vi "tcp_echo_client.vi"() -> ()   [LabVIEW 2015]
panel:
  out "good echo":bool
  out "message received":string
  in  "message to send":string="hello there.\r\n"
  out "available IP addresses":string[](array[string])
  in  "remote port or service name":u16=7
  in  "address":string
  # "try tcp ping"
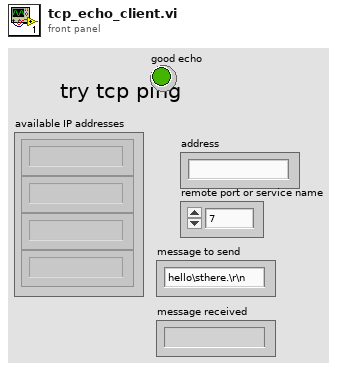
[diagram p1: front panel]
types:
  T1 = enum16{"Standard", "Buffered", "CRLF", "Immediate"}
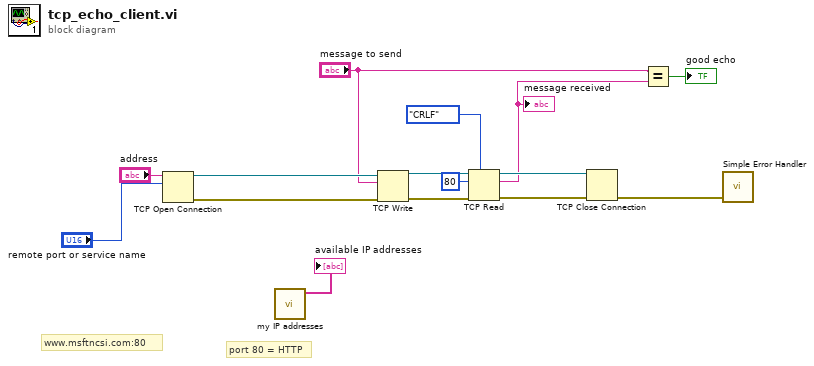
[diagram p0: block diagram]
diagram:
  # "port 80 = HTTP"
  # "www.msftncsi.com:80"
  n1 = TCP Open Connection(address="address", remote port or service name="remote port or service name") -> (connection ID=w4:refnum<k5>, error out=w5:errorcluster)  [unwired: 3 in]
  n2 = call "my IP addresses.vi"() -> ("available IP addresses"=→"available IP addresses":string[])  [unwired: 10 in, 1 out]
  n3 = TCP Write(connection ID=w4, data in="message to send", error in (no error)=w5) -> (connection ID out=w11:refnum<k5>, error out=w12:errorcluster)  [unwired: 1 in, 1 out]
  n4 = TCP Read(connection ID=w11, bytes to read=80, error in (no error)=w12, 7:T1."CRLF" ("mode (standard)")) -> (connection ID out=w8:refnum<k5>, data out=w3:string, error out=w9:errorcluster)  [unwired: 1 in]
  "message received" <- w3
  n5 = TCP Close Connection(connection ID=w8, error in (no error)=w9) -> (error out=w7:errorcluster)  [unwired: 1 in, 1 out]
  n6 = Equal?(x="message to send", y=w3) -> (x = y?=→"good echo":bool)
  n7 = call <vilib>:"Simple Error Handler.vi"("error in (no error)"=w7) -> ()  [unwired: 4 in, 5 out]
